vi "test_DiscoveryWrapper_StopDiscoveryService_WrapperMethodsWorkWithoutError.vi"(8 "error in":errorcluster) -> (0 "error out":errorcluster, 2 "result":string, 3 "pass":bool)   [LabVIEW 2020, in "MeasurementServerTests.lvlib" / "Discovery Tests.lvlib"]
uses:
  Discovery Tests.lvlib
  Runtime/MeasurementLink Discovery Client/RPC Messages/ni_measurementlink_discovery_v1_ResolveServiceRequest.ctl
  MeasurementServerTests.lvlib
  Runtime/MeasurementLink Discovery V1/MeasurementLink Discovery V1.lvlib
  Runtime/MeasurementLink Discovery Client/MeasurementLink Discovery Client.lvlib
panel:
  in  "file (use dialog)":path=path "C:/info.txt"
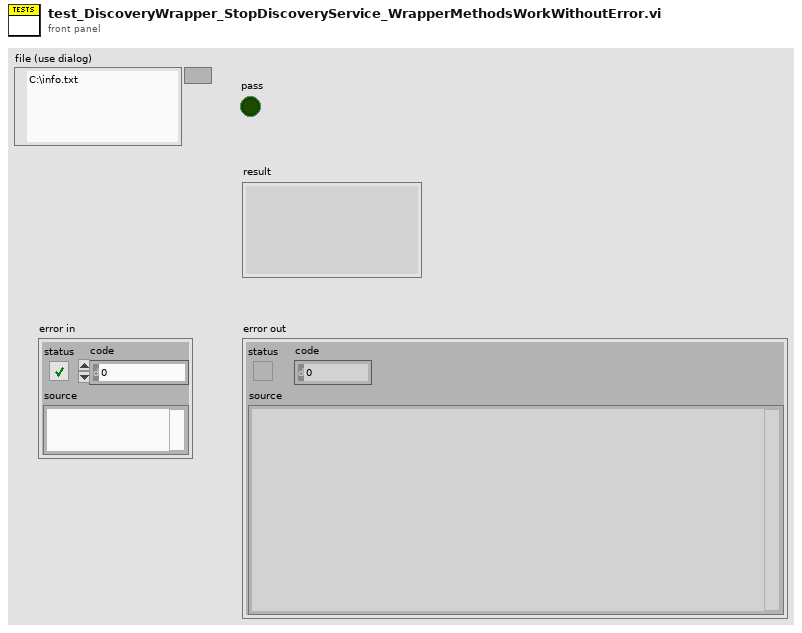
[diagram p1: front panel]
types:
  T1 = typedef "MeasurementLink Discovery Client.lvlib/ni_measurementlink_discovery_v1_ResolveServiceRequest.ctl" = cluster{"provided_interface":string, "service_class":string}
  T2 = typedef "MeasurementLink Discovery Client.lvlib/ni_measurementlink_discovery_v1_ServiceLocation.ctl" = cluster{"location":string, "insecure_port":string, "ssl_authenticated_port":string}
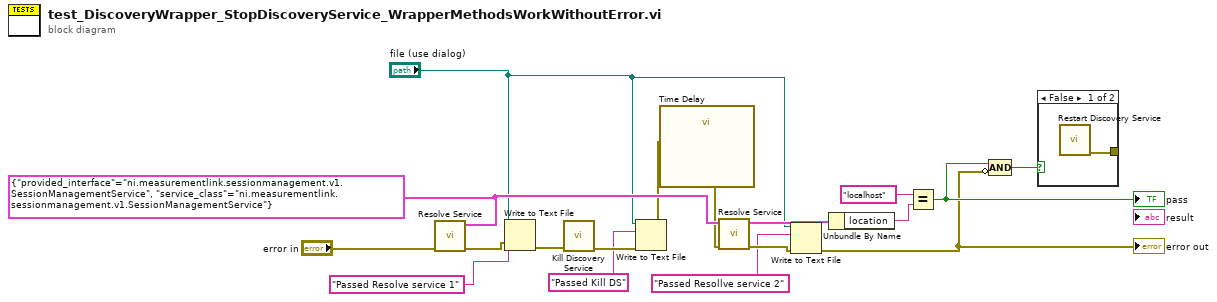
[diagram p0: block diagram]
diagram:
  w12 = T1 {"provided_interface"="ni.measurementlink.sessionmanagement.v1.SessionManagementService", "service_class"="ni.measurementlink.sessionmanagement.v1.SessionManagementService"} ("request data")
  n1 = call "Resolve Service.vi"("error in"="error in", "request data"=w12) -> ("error out"=w4:errorcluster)  [unwired: 8 in, 1 out]
  n2 = Write to Text File(file (use dialog)="file (use dialog)", text="Passed Resolve service 1", error in=w4) -> (error out=w3:errorcluster)  [unwired: 1 in, 2 out]
  n3 = call "Kill Discovery Service.vi"("error in"=w3) -> ("error out"=w10:errorcluster)  [unwired: 10 in]
  n4 = Write to Text File(file (use dialog)="file (use dialog)", text="Passed Kill DS", error in=w10) -> (error out=w2:errorcluster)  [unwired: 1 in, 2 out]
  n5 = call "Time Delay"("error in (no error)"=w2) -> ("error out"=w1:errorcluster)  [unwired: 10 in]
  n6 = call "Resolve Service.vi"("error in"=w1, "request data"=w12) -> ("error out"=w8:errorcluster, "response data"=w17:T2)  [unwired: 8 in]
  n7 = Write to Text File(file (use dialog)="file (use dialog)", text="Passed Resollve service 2", error in=w8) -> (error out=w7:errorcluster)  [unwired: 1 in, 2 out]
  "error out" <- w7
  n8 = Unbundle By Name(w17) -> ("location"=w16:string)
  n9 = Equal?(x="localhost", y=w16) -> (x = y?=w15:bool)
  "pass" <- w15
  n10 = Compound Arithmetic op=AND(w15, invert w7) -> (w18:bool)
  n11 = case shown="False" w18 {
    tunnel: [w19 _] -> _
    frame False {
      n12 = call "Restart Discovery Service.vi"() -> ("error out"=w19:errorcluster)  [unwired: 11 in]
    }
    frame True {
    }
  }
